vi "Get Process Memory Info x64.vi"(8 "error in (no error)":errorcluster) -> (0 "error out":errorcluster, 3 "ppsmemCounters":T1)   [LabVIEW 2017]
uses:
  kernel32.dll
  psapi.dll
panel:
  out "return type":u64
  out "x/y":dbl
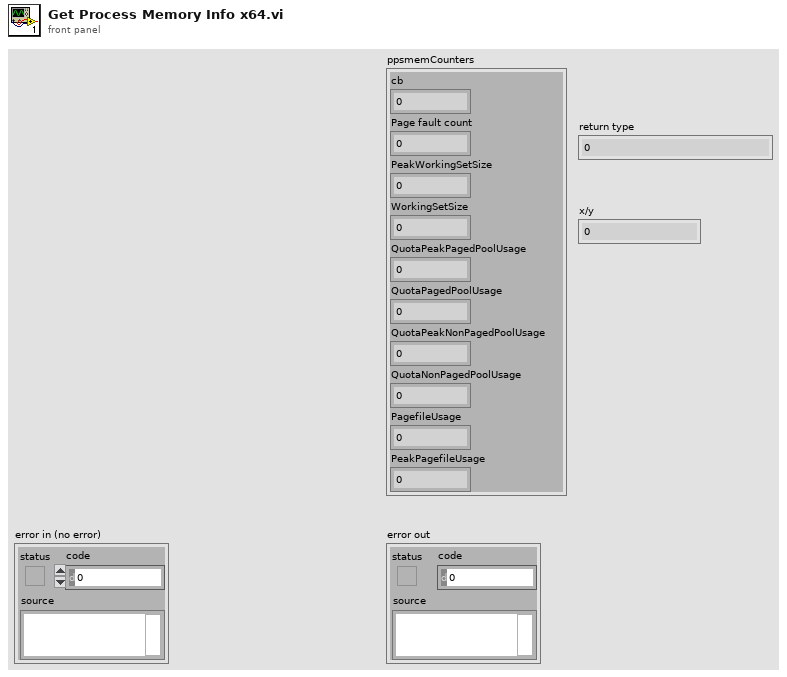
[diagram p1: front panel]
types:
  T1 = cluster{"cb":u32, "Page fault count":u32, "PeakWorkingSetSize":u64, "WorkingSetSize":u64, "QuotaPeakPagedPoolUsage":u64, "QuotaPagedPoolUsage":u64, "QuotaPeakNonPagedPoolUsage":u64, "QuotaNonPagedPoolUsage":u64, "PagefileUsage":u64, "PeakPagefileUsage":u64}
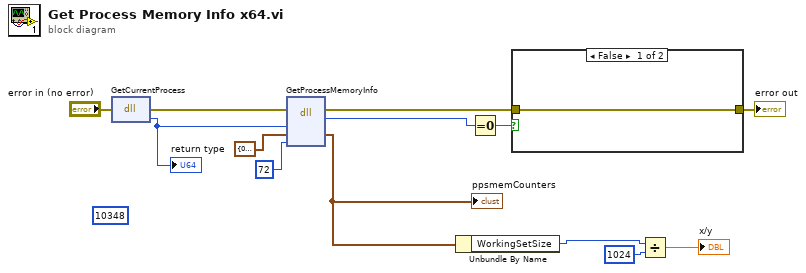
[diagram p0: block diagram]
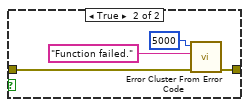
[diagram p2: hidden frame]
diagram:
  (unwired) u64 10348 ("Process")
  n1 = dll-call lib="kernel32.dll" fn="GetCurrentProcess"(error in="error in (no error)") -> (error out=w13:errorcluster, "return type"=w1:u64)  [unwired: 2 in, 1 out]
  "return type" <- w1
  n2 = dll-call lib="Psapi.dll" fn="GetProcessMemoryInfo"(error in=w13, "Process"=w1, "ppsmemCounters"=T1 {"cb"=0, "Page fault count"=0, "PeakWorkingSetSize"=0, "WorkingSetSize"=0, "QuotaPeakPagedPoolUsage"=0, "QuotaPagedPoolUsage"=0, "QuotaPeakNonPagedPoolUsage"=0, "QuotaNonPagedPoolUsage"=0, "PagefileUsage"=0, "PeakPagefileUsage"=0} ("Cluster"), "cb"=u32 72) -> (error out=w6:errorcluster, "return type"=w10:i32, "ppsmemCounters"=w5:T1)  [unwired: 4 in, 1 out]
  "ppsmemCounters" <- w5
  n3 = Unbundle By Name(w5) -> ("WorkingSetSize"=w3:u64)
  n4 = Equal To 0?(x=w10) -> (x = 0?=w9:bool)
  n5 = case shown="False" w9 {
    tunnel: w6 -> [w14 w18]
    tunnel: [w14 w17] -> w8
    frame False {
    }
    frame True {
      n6 = call <vilib>:"Error Cluster From Error Code.vi"("error in (no error)"=w18, "error message (\"\")"="Function failed." ("error message (\"\")"), "error code (0)"=5000) -> ("error out"=w17:errorcluster)  [unwired: 6 in]
    }
  }
  "error out" <- w8
  n7 = Divide(x=w3, y=u32 1024) -> (x/y=→"x/y":dbl)
